vi "FPGA Time Management.vi"   [LabVIEW 2023]
uses:
  <vilib>/Platform/TimedLoop/XDataNode/timing_clust.ctl
  <vilib>/Platform/TimedLoop/XDataNode/nitl_modes.ctl
  <vilib>/Platform/TimedLoop/XDataNode/wakeup.ctl
  <vilib>/rvi/Emulation/niFpgaGetClockAttributes.vi
  <vilib>/rvi/Emulation/niFpgaSctlEmulationGetInTimedLoop.vi
  <vilib>/rvi/Emulation/niFpgaEmulationReportErrorSimple.vi
  <vilib>/rvi/eio/common/nirviEmuTemplateMethod_errors.vi
  Front Panel Globals.vi
  <vilib>/rvi/Emulation/niFpgaProcessEmulError.vi
  <vilib>/rvi/eio/common/nirviEmuTemplatePropertyGet_noerrors.vi
  <vilib>/rvi/Emulation/niFpgaCriticalErrorInLSC.vi
  <vilib>/eio/EIOMethodNode/EIOMethodNode.xnode
  <vilib>/eio/EIOPropertyNode/EIOPropertyNode.xnode
  <vilib>/LabVIEW Targets/FPGA/cRIO/shared/nicrio_ModuleControls/nicrio_cRIO-9467_Latitude.ctl
  <vilib>/LabVIEW Targets/FPGA/cRIO/shared/nicrio_ModuleControls/nicrio_cRIO-9467_Longitude.ctl
  <vilib>/LabVIEW Targets/FPGA/cRIO/shared/nicrio_ModuleControls/nicrio_cRIO-9467_Altitude.ctl
  <vilib>/eio/EIONode/EIONode.xnode
  <vilib>/platform/TimedLoop/XDataNode/XDataNode.xnode
  FPGA Timekeeper 1.1b0/FPGA Timekeeper.lvlib
  <vilib>/rvi/eio/common/nirviEmuTemplatePropertyGet_errors.vi
  <vilib>/rvi/eio/common/nirviEmuTemplatePropertySet_errors.vi
  <vilib>/rvi/eio/common/nirviEmuTemplatePropertySet_noerrors.vi
  <vilib>/Platform/TimedLoop/XDataNode/XDNodeRunTimeDep.lvlib
types:
  T1 = enum8{"Initializing", "Normal", "Unable to get fix"}
  T2 = enum8{"Unknown", "Normal", "Absent", "Overcurrent"}
  T3 = typedef "nicrio_cRIO-9467_Latitude.ctl" = fxp<+/-,28,8>
  T4 = typedef "nicrio_cRIO-9467_Longitude.ctl" = fxp<+/-,29,9>
  T5 = typedef "nicrio_cRIO-9467_Altitude.ctl" = fxp<+/-,24,17>
  T6 = typedef "XDNodeRunTimeDep.lvlib/timing_clust.ctl" = cluster{"Expected End [f-1]":u64, "Actual End [f-1]":u64, "Finished Late? [f-1]":bool, "Expected End [i-1]":u64, "Actual End [i-1]":u64, "Finished Late? [i-1]":bool, "Expected Start [i]":u64, "Actual Start [i]":u64, "Expected Start [f]":u64, "Actual Start [f]":u64, "Source Name":string, "Structure Name":string, "Period":i64, "Deadline":i64, "Offset":i64, "Start":i64, "Priority":i32, "Timeout":i32, "Mode":T7, "Wakeup Reason":T8, "Error":errorcluster, "Source Type":string, "Secondary Source Type":string, "Global End Time":u64, "Global Start Time":u64, "Frame Duration":u64, "Iteration Duration":u64, "Assigned CPU":i32, "I/O Scan Engine Mode":u32}
  T7 = typedef "XDNodeRunTimeDep.lvlib/nitl_modes.ctl" = enum32{"No Change", "Process missed periods, maintain original phase", "Discard missed periods, maintain original phase", "Process missed periods, ignore original phase", "Discard missed periods, ignore original phase"}
  T8 = typedef "XDNodeRunTimeDep.lvlib/wakeup.ctl" = enum32{"Normal", "Aborted", "Asynchronous wakeup", "Timing source error", "Timed loop error", "Timeout"}
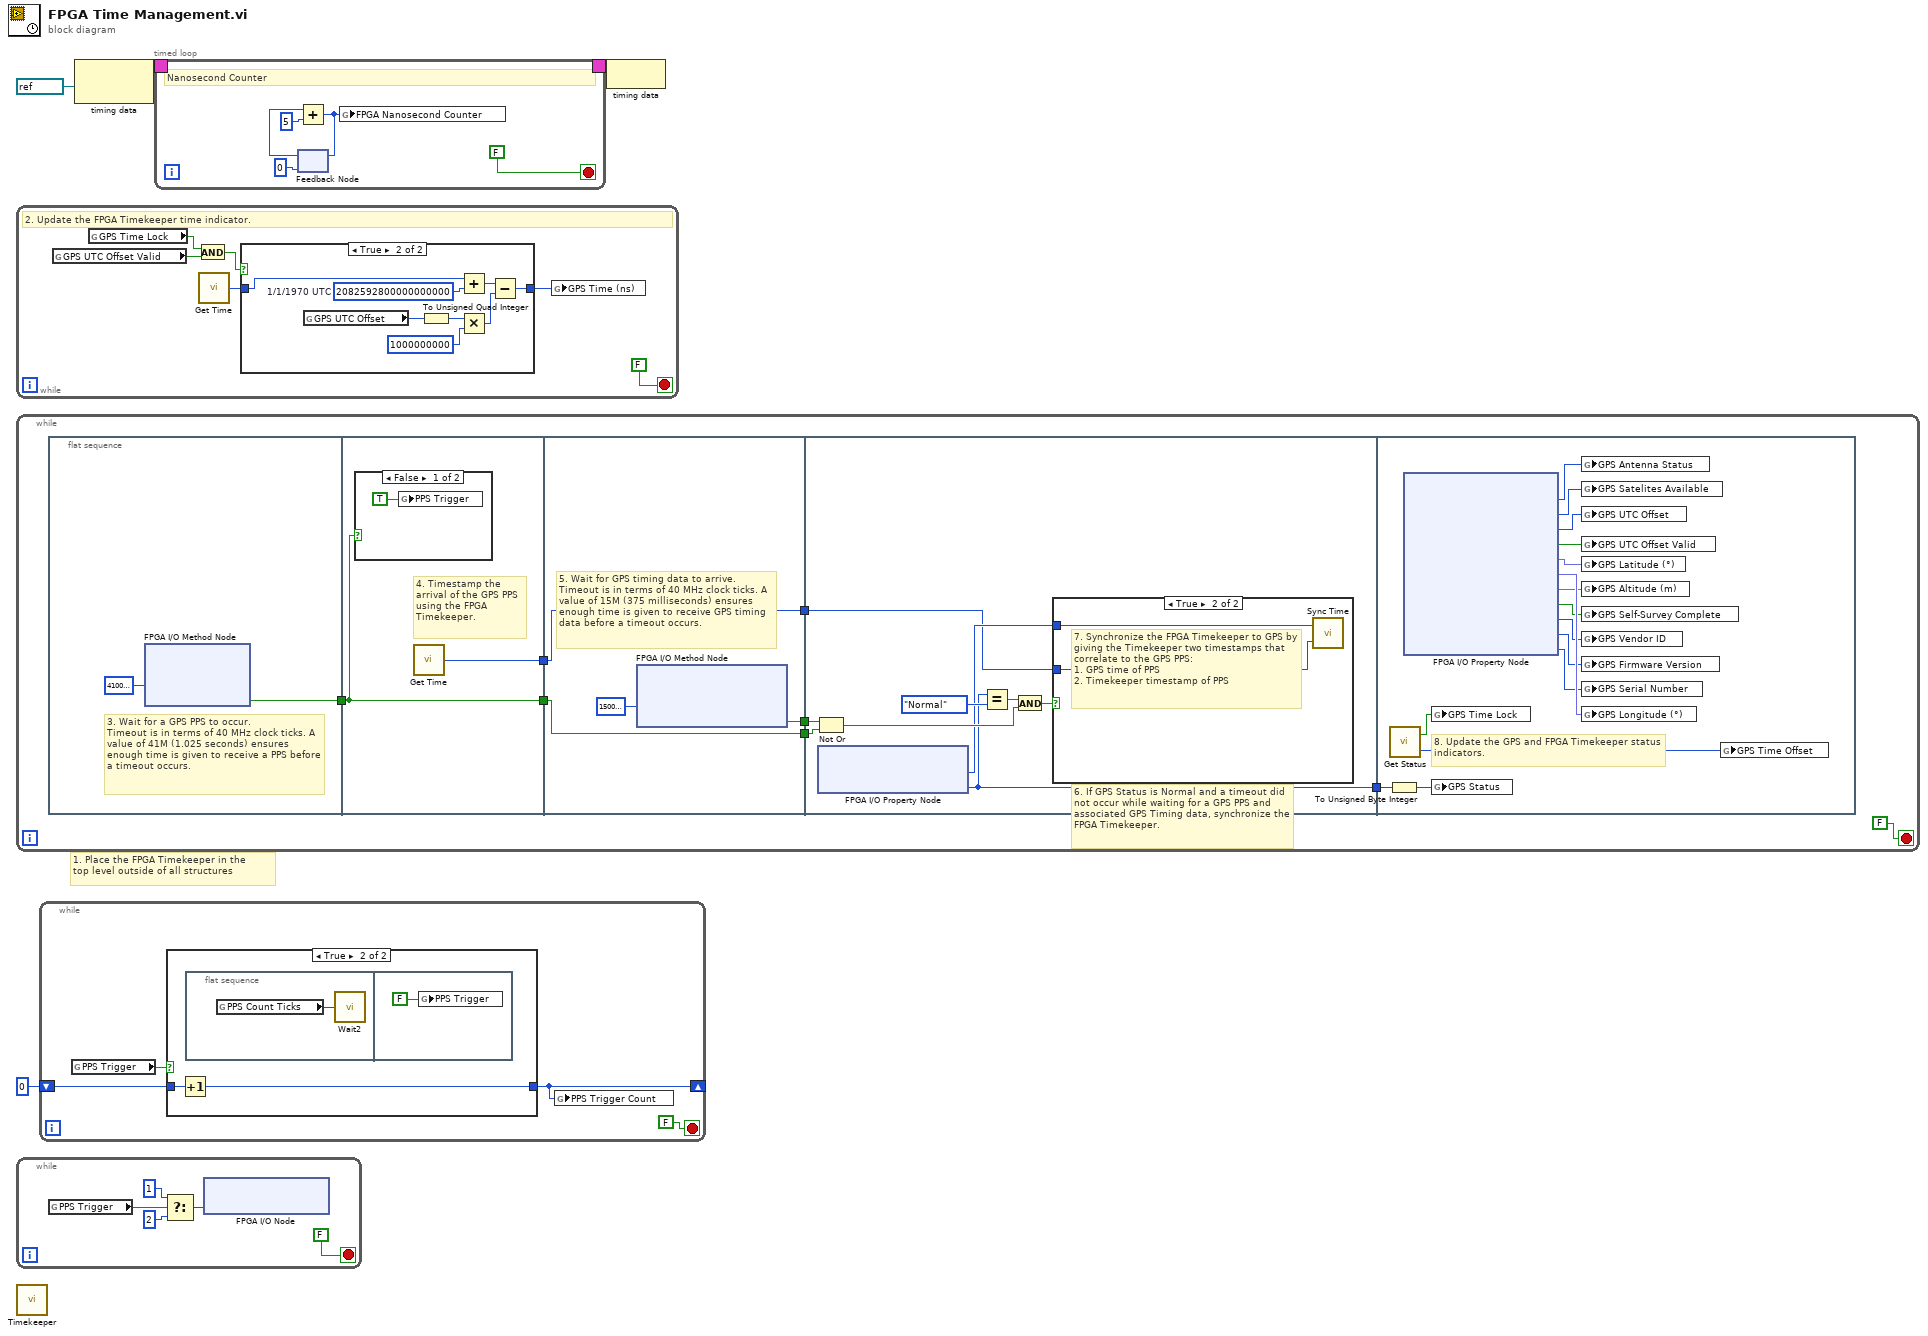
[diagram p0: block diagram]
diagram:
  # "1. Place the FPGA Timekeeper in the\ntop level outside of all structures"
  n1 = while {
    stop <- FALSE stop-if-true
    # "2. Update the FPGA Timekeeper time indicator."
    n2 = global read "Front Panel Globals.vi" "GPS UTC Offset Valid"() -> (w6:bool)
    n3 = global read "Front Panel Globals.vi" "GPS Time Lock"() -> (w7:bool)
    n4 = And(x=w7, y=w6) -> (x .and. y?=w5:bool)
    n5 = call "Get Time.vi"() -> ("time (ns)"=w9:u64)
    n6 = case shown="True" w5 {
      tunnel: w9 -> [w11 w19]
      tunnel: [w11 w13] -> w8
      frame False {
      }
      frame True {
        w12 = u64 2082592800000000000  # 1/1/1970 UTC
        n7 = global read "Front Panel Globals.vi" "GPS UTC Offset"() -> (w18:i8)
        n8 = To Unsigned Quad Integer(1:w18) -> (0:w17:u64)
        n9 = Add(x=w19, y=w12) -> (x+y=w15:u64)
        n10 = Multiply(x=w17, y=u64 1000000000) -> (x*y=w14:u64)
        n11 = Subtract(x=w15, y=w14) -> (x-y=w13:u64)
      }
    }
    n12 = global write "Front Panel Globals.vi" "GPS Time (ns)"(w8) -> ()
  }
  n13 = while {
    stop <- FALSE stop-if-true
    n14 = flat-sequence {
      tunnel: [w28] -> w26
      tunnel: w26 -> [w30]
      tunnel: [w30] -> w25
      tunnel: [w31] -> w23
      tunnel: [w35] -> w27
      tunnel: w25 -> [w34]
      tunnel: [w34] -> w24
      tunnel: w23 -> [w33]
      tunnel: [w33] -> w22
      tunnel: w27 -> [w44]
      tunnel: w24 -> [w43]
      tunnel: w22 -> [w38]
      tunnel: [w37] -> w21
      tunnel: w21 -> [w62]
      frame #0 {
        # "3. Wait for a GPS PPS to occur.\nTimeout is in terms of 40 MHz clock ticks. A value of 41M (1.025 seconds) ensures enough time is given to receive a PPS before a timeout occurs."
        n15 = xnode "FPGA I/O Method Node"("Timeout"=41000000) -> ("Timed Out"=w28:bool)  [unwired: 1 in, 1 out]
      }
      frame #1 {
        # "4. Timestamp the arrival of the GPS PPS using the FPGA Timekeeper."
        n16 = case shown="False" w30 {
          frame False {
            n17 = global write "Front Panel Globals.vi" "PPS Trigger"(TRUE ("PPS Trigger")) -> ()
          }
          frame True {
          }
        }
        n18 = call "Get Time.vi"() -> ("time (ns)"=w31:u64)
      }
      frame #2 {
        # "5. Wait for GPS timing data to arrive.\nTimeout is in terms of 40 MHz clock ticks. A value of 15M (375 milliseconds) ensures enough time is given to receive GPS timing data before a timeout occurs."
        n19 = xnode "FPGA I/O Method Node"("Timeout"=15000000) -> ("Timed Out"=w35:bool)  [unwired: 1 in, 1 out]
      }
      frame #3 {
        # "6. If GPS Status is Normal and a timeout did not occur while waiting for a GPS PPS and associated GPS Timing data, synchronize the FPGA Timekeeper."
        n20 = Not Or(1:w43, 2:w44) -> (0:w41:bool)
        n21 = xnode "FPGA I/O Property Node"() -> ("PPS Timestamp (TAI)"=w39:u64, "GPS Status"=w37:T1)  [unwired: 1 in, 1 out]
        n22 = Equal?(x=w37, y=T1."Normal") -> (x = y?=w42:bool)
        n23 = And(x=w42, y=w41) -> (x .and. y?=w40:bool)
        n24 = case shown="True" w40 {
          tunnel: w39 -> [_ w47]
          tunnel: w38 -> [_ w46]
          frame False {
          }
          frame True {
            # "7. Synchronize the FPGA Timekeeper to GPS by giving the Timekeeper two timestamps that correlate to the GPS PPS:\n1. GPS time of PPS\n2. Timekeeper timestamp of PPS"
            n25 = call "Sync Time.vi"("FPGA Timekeeper time (ns)"=w46, "time reference time (ns)"=w47) -> ()
          }
        }
      }
      frame #4 {
        # "8. Update the GPS and FPGA Timekeeper status indicators."
        n26 = To Unsigned Byte Integer(number=w62) -> (unsigned 8bit integer=w55:u8)
        n27 = call "Get Status.vi"() -> ("FPGA Timekeeper locked"=w60:bool, "offset from time reference"=w61:i32)
        n28 = xnode "FPGA I/O Property Node"() -> ("Antenna Status"=w56:T2, "Satellites Available"=w57:u8, "UTC Offset"=w58:i8, "UTC Offset Valid"=w59:bool, "Latitude (°)"=w54:T3, "Longitude (°)"=w53:T4, "Altitude (m)"=w52:T5, "Self-Survey Complete"=w49:bool, "Vendor ID"=w51:u16, "Firmware Version"=w50:u32, "Serial Number"=w48:u32)  [unwired: 1 in, 1 out]
        n29 = global write "Front Panel Globals.vi" "GPS Time Lock"(w60) -> ()
        n30 = global write "Front Panel Globals.vi" "GPS Status"(w55) -> ()
        n31 = global write "Front Panel Globals.vi" "GPS Antenna Status"(w56) -> ()
        n32 = global write "Front Panel Globals.vi" "GPS Satelites Available"(w57) -> ()
        n33 = global write "Front Panel Globals.vi" "GPS UTC Offset"(w58) -> ()
        n34 = global write "Front Panel Globals.vi" "GPS UTC Offset Valid"(w59) -> ()
        n35 = global write "Front Panel Globals.vi" "GPS Latitude (°)"(w54) -> ()
        n36 = global write "Front Panel Globals.vi" "GPS Altitude (m)"(w52) -> ()
        n37 = global write "Front Panel Globals.vi" "GPS Self-Survey Complete"(w49) -> ()
        n38 = global write "Front Panel Globals.vi" "GPS Vendor ID"(w51) -> ()
        n39 = global write "Front Panel Globals.vi" "GPS Firmware Version"(w50) -> ()
        n40 = global write "Front Panel Globals.vi" "GPS Serial Number"(w48) -> ()
        n41 = global write "Front Panel Globals.vi" "GPS Longitude (°)"(w53) -> ()
        n42 = global write "Front Panel Globals.vi" "GPS Time Offset"(w61) -> ()
      }
    }
  }
  n43 = while {
    stop <- FALSE stop-if-true
    n44 = global read "Front Panel Globals.vi" "PPS Trigger"() -> (w67:bool)
    n45 = Select(t=u8 1 ("USER FPGA LED"), s=w67, f=u8 2 ("USER FPGA LED")) -> (s? t:f=w64:u8)
    n46 = xnode "FPGA I/O Node"("USER FPGA LED"=w64) -> ()  [unwired: 1 in, 1 out]
  }
  n47 = call "Timekeeper.vi"() -> ()  [unwired: 12 in]
  n48 = while {
    shift-right: [w68] -> _
    shift-left: u32 0 -> [w69]
    stop <- FALSE stop-if-true
    n49 = global read "Front Panel Globals.vi" "PPS Trigger"() -> (w70:bool)
    n50 = case shown="True" w70 {
      tunnel: [w72 w74] -> w68
      tunnel: w69 -> [w72 w73]
      frame False {
      }
      frame True {
        n51 = Increment(x=w73) -> (x+1=w74:u32)
        n52 = flat-sequence {
          frame #0 {
            n53 = global read "Front Panel Globals.vi" "PPS Count Ticks"() -> (w75:u32)
            n54 = call "Wait2"("Count(Ticks)"=w75) -> ()  [unwired: 1 out]
          }
          frame #1 {
            n55 = global write "Front Panel Globals.vi" "PPS Trigger"(FALSE ("PPS Trigger")) -> ()
          }
        }
      }
    }
    n56 = global write "Front Panel Globals.vi" "PPS Trigger Count"(w68) -> ()
  }
  n57 = node-c288(refnum<k21> "200MHz" ("Source Name")) -> (w4:T6)
  n58 = timed-loop {
    timing: w4 -> [_]
    timing-out: [_] -> w3
    stop <- FALSE stop-if-true
    # "Nanosecond Counter"
    n59 = feedback #1(u64 0) -> (w80:u64)
    n60 = Add(x=w80, y=u64 5) -> (x+y=w77:u64)
    n61 = feedback-in #1(w77) -> ()
    n62 = global write "Front Panel Globals.vi" "FPGA Nanosecond Counter"(w77) -> ()
  }
  n63 = node-c288(w3) -> ()
